vi "Follow Path Single Side.vi"(0 "segments":T1, 1 "output range":cluster{"output high":dbl, "output low":dbl}={"output high"=1.0, "output low"=-1.0} {"output low" format="%.2f"; "output high" format="%.2f"}, 2 "invert? (F)":bool, 5 "Encoder":dbl format="%.2f", 7 "Kv":dbl, 9 "Ka":dbl, 11 "i Zone":dbl=inf format="%.2f", 12 "PIDF gains":cluster{"Kp":dbl, "Ki":dbl, "Kd":dbl, "Kf":dbl} {"Kf" format="%.3f"; "Kd" format="%.3f"; "Ki" format="%.3f"; "Kp" format="%.3f"}, 13 "reinitialize? (F)":bool) -> (4 "output":dbl)   [LabVIEW 2016, in "Drive System.lvlib"]
uses:
  Drive System.lvlib
  Pathfinder/VIs/Segment.ctl
  Pathfinder/Pathfinder.lvlib
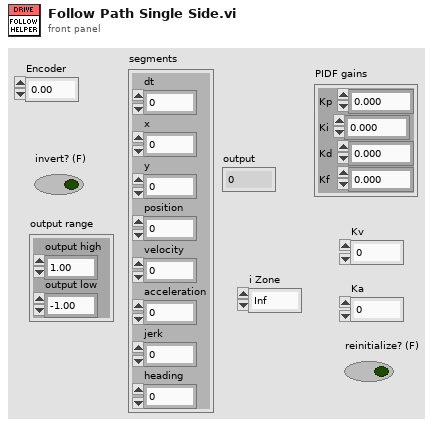
[diagram p1: front panel]
types:
  T1 = typedef "Pathfinder.lvlib/Segment.ctl" = cluster{"dt":dbl, "x":dbl, "y":dbl, "position":dbl, "velocity":dbl, "acceleration":dbl, "jerk":dbl, "heading":dbl}
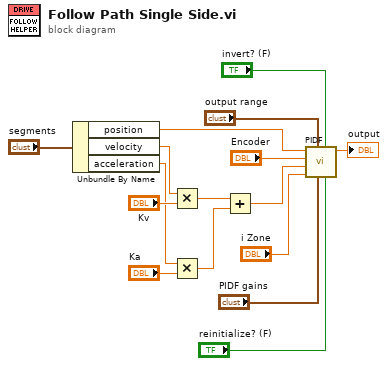
[diagram p0: block diagram]
diagram:
  n1 = Unbundle By Name("segments") -> ("position"=w4:dbl, "velocity"=w3:dbl, "acceleration"=w2:dbl)
  n2 = Multiply(x=w3, y="Kv") -> (x*y=w6:dbl)
  n3 = Multiply(x=w2, y="Ka") -> (x*y=w7:dbl)
  n4 = Add(x=w6, y=w7) -> (x+y=w8:dbl)
  n5 = call "PIDF.vi"("reinitialize? (F)"="reinitialize? (F)", "invert? (F)"="invert? (F)", "PIDF gains"="PIDF gains", "output range"="output range", "i Zone"="i Zone", "Feedforward"=w8, "process variable"="Encoder", "setpoint"=w4) -> ("output"=→"output":dbl)  [unwired: 3 in]
